vi "Set slit width.vi"(8 "error in (no error)":errorcluster, 11 "DAQOrcaFlash in":refnum<class "DAQOrcaFlash.lvclass">) -> (0 "error out":errorcluster, 3 "DAQOrcaFlash out":refnum<class "DAQOrcaFlash.lvclass">)   [LabVIEW 2012, in "DAQOrcaFlash.lvclass"]
uses:
  DAQOrcaFlash.lvclass
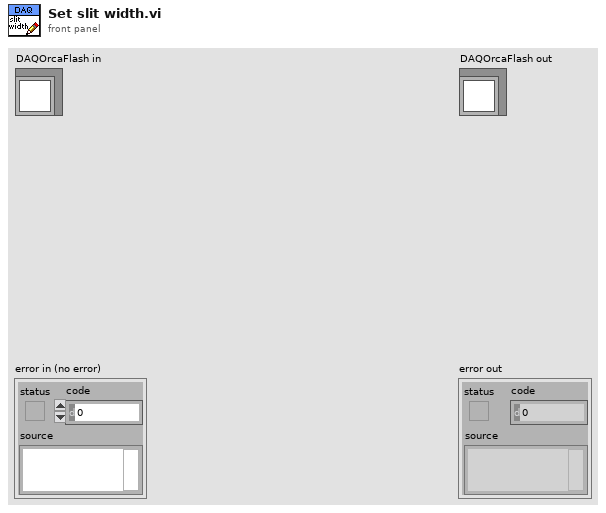
[diagram p1: front panel]
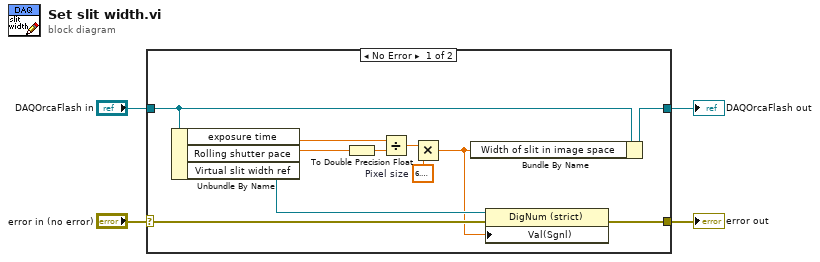
[diagram p0: block diagram]
diagram:
  n1 = case shown="No Error" "error in (no error)" {
    selector: "error in (no error)" -> [w10 w17]
    tunnel: [w9 w17] -> w3
    tunnel: [w11 w16] -> w1
    tunnel: "DAQOrcaFlash in" -> [w12 w16]
    frame No Error {
      w13 = dbl[unit] 6.5e-06  # Pixel size
      n2 = Unbundle By Name(w12) -> ("exposure time"=w15:dbl[unit], "Rolling shutter pace"=w5:sgl[unit], "Virtual slit width ref"=w8:refnum<vi>)
      n3 = To Double Precision Float(number=w5) -> (double precision float=w6:dbl[unit])
      n4 = Divide(x=w15, y=w6) -> (x/y=w14:dbl)
      n5 = Multiply(x=w14, y=w13) -> (x*y=w7:dbl[unit])
      n6 = Bundle By Name(cluster=w12, "Width of slit in image space"=w7) -> (w11:refnum<class "DAQOrcaFlash.lvclass">)
      n7 = property class="DigNum (strict)"(reference=w8, error in=w10, "Val(Sgnl)"=w7) -> (error out=w9:errorcluster)  [unwired: 1 out]
    }
    frame Error {
    }
  }
  "error out" <- w3
  "DAQOrcaFlash out" <- w1
